vi "WriteB (SubVI).vi"(7 "Try":i32=5, 8 "error IO":errorcluster, 9 "Sweep rate":dbl=0.1, 10 "Target B":dbl, 11 "VISA resource name":refnum<visa-resource-name>) -> (0 "error out":errorcluster, 3 "VISA Refnum out":refnum<visa-resource-name>)   [LabVIEW 2016]
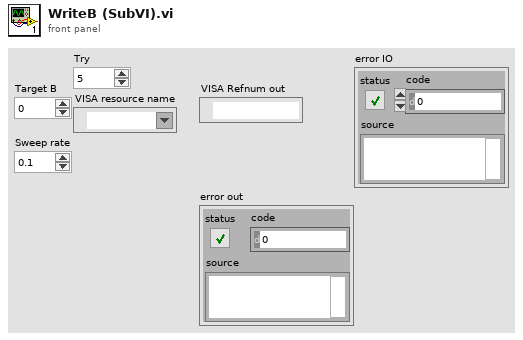
[diagram p1: front panel]
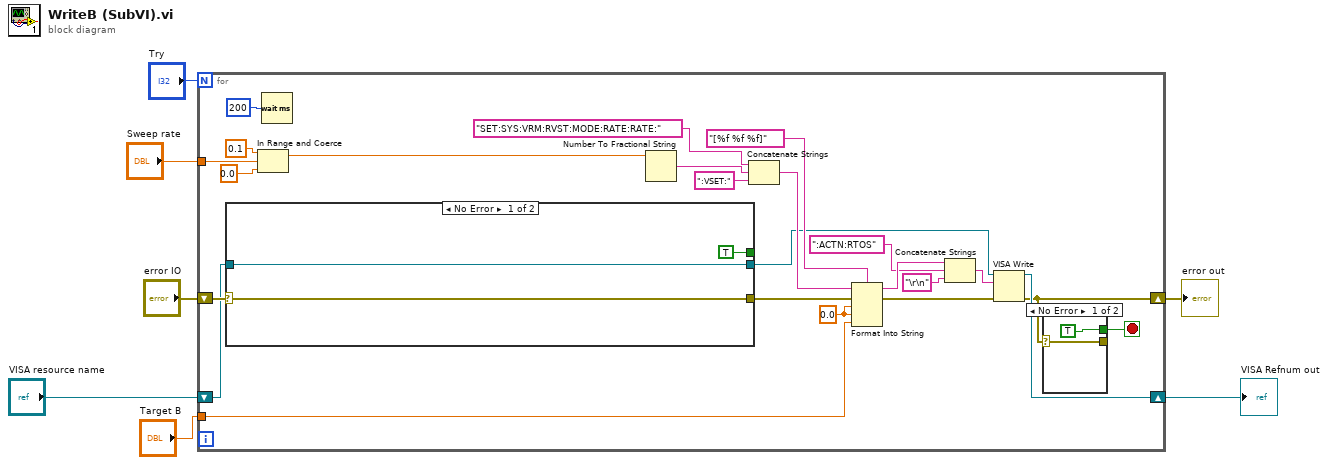
[diagram p0: block diagram]
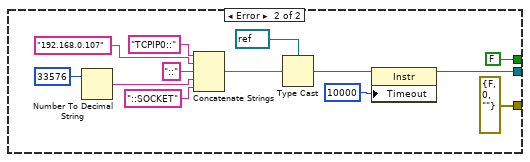
[diagram p2: hidden frame]
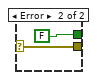
[diagram p3: hidden frame]
diagram:
  n1 = for {
    N: "Try" -> [_]
    tunnel: "Target B" -> [w31]
    tunnel: "Sweep rate" -> [w11]
    shift-right: [w14] -> w2
    shift-left: "error IO" -> [w19]
    shift-right: [w16] -> w5
    shift-left: "VISA resource name" -> [w18]
    stop <- w13 stop-if-true
    w21 = 0.0
    n2 = case shown="No Error" w19 {
      selector: w19 -> [w34 _]
      tunnel: [w34 errorcluster {"status"=FALSE, "code"=0, "source"=""} ("error IO")] -> w15
      tunnel: [w33 w37] -> w17
      tunnel: w18 -> [w33 _]
      tunnel: [TRUE FALSE] -> _
      frame No Error {
      }
      frame Error {
        n3 = Number To Decimal String(number=33576 ("Port")) -> (decimal integer string=w42:string)  [unwired: 1 in]
        n4 = Concatenate Strings("TCPIP0::" ("string"), "192.168.0.107" ("IP address"), "::" ("string"), w42, "::SOCKET" ("string")) -> (w40:string)
        n5 = Type Cast(type=refnum<visa-resource-name> refnum ("VISA resource name"), x=w40) -> (*(type *) &x=w39:refnum<visa-resource-name>)
        n6 = property class="Instr"(reference=w39, "Timeout"=u32 10000 ("General Settings:Timeout Value")) -> (reference out=w37:refnum<visa-resource-name>)  [unwired: 1 in, 1 out]
      }
    }
    n7 = In Range and Coerce(upper limit=0.1, x=w11, lower limit=0.0) -> (coerced(x)=w8:dbl)  [unwired: 1 out]
    n8 = Wait (ms)(milliseconds to wait=u32 200) -> ()  [unwired: 1 out]
    n9 = Number To Fractional String(number=w8) -> (F-format string=w23:string)  [unwired: 3 in]
    n10 = Concatenate Strings("SET:SYS:VRM:RVST:MODE:RATE:RATE:", w23, ":VSET:") -> (w22:string)
    n11 = Format Into String(format string="[%f %f %f]", initial string=w22, error in=w15, w21, w21, w31) -> (resulting string=w28:string, error out=w30:errorcluster)
    n12 = Concatenate Strings(w28, ":ACTN:RTOS", "\r\n" ("string")) -> (w29:string)
    n13 = VISA Write(VISA resource name=w17, write buffer=w29, error in (no error)=w30) -> (VISA resource name out=w16:refnum<visa-resource-name>, error out=w14:errorcluster)  [unwired: 1 out]
    n14 = case shown="No Error" w14 {
      selector: w14 -> [w49 w51]
      tunnel: [w49 w51] -> _
      tunnel: [TRUE FALSE] -> w13
      frame No Error {
      }
      frame Error {
      }
    }
  }
  "VISA Refnum out" <- w5
  "error out" <- w2
